vi "CAN User Interface.vi"() -> ()   [LabVIEW 2023, in "GUI.lvlib" / "Diagnostic.lvlib"]
uses:
  Diagnostic.lvlib
  Teststand Steptypes/CAN/STP/Steptypes/Control/STP Data.ctl
  HardwareAbstractionLayer_LVOOP/CAN/CAN Application Protocols/STP Protocol_class/Ctrls/STP CMD.ctl
  Teststand Steptypes/CAN/STP/Steptypes/Control/STP Out Data.ctl
  HardwareAbstractionLayer_LVOOP/CAN/CAN Application Protocols/STP Protocol_class/Ctrls/STP Error Cluster.ctl
  HardwareAbstractionLayer_LVOOP/CAN/CAN Lib/Control/CAN Table.ctl
  HardwareAbstractionLayer_LVOOP/Database/SQL Public VI/Control/DB Options.ctl
  HardwareAbstractionLayer_LVOOP/Database/Database.lvclass
  HardwareAbstractionLayer_LVOOP/CAN/CAN Lib/CAN HAL Lib.lvlib
  HardwareAbstractionLayer_LVOOP/CAN/CAN Application Protocols/STP Protocol_class/STP Protocol.lvclass
  Teststand Steptypes/LTT_TeststandSteptypes.lvlib
panel:
  in  "Socket No":u16=1
  in  "Clear":bool=TRUE
  in  "Log Data?":bool=TRUE
  out "error out":errorcluster
  in  "error in":errorcluster
  in  "Tab Control":enum32{"Query", "Logs"}(tab)
  in  "STP Data in":T1={"ECU CAN Port"="CAN1", "CMD"=130, "CAN Write Data"=[], "Response Decoder"=enum."String", "String"={"Start Index"=0, "Length"=-1}, "Number"={"MSB Index"=0, "LSB Index"=1}, "Boolean"={"Index"=0, "Bool"={"7"=FALSE, "6"=FALSE, "5"=FALSE, "4"=FALSE, "3"=FALSE, "2"=FALSE, "1"=FALSE, "0"=FALSE, "7 Enabled"=FALSE, "6 Enabled"=FALSE, "5 Enabled"=FALSE, "4 Enabled"=FALSE, "3 Enabled"=FALSE, "2 Enabled"=FALSE, "1 Enabled"=FALSE, "0 Enabled"=FALSE}}} {"CMD" items=["TSW_VERSION(130)"=130, "WAIT_EVENT(132)"=132, "SEQUENCER(133)"=133, "TSW_RESET(150)"=150, "CONFIG_ECU(151)"=151, "TEST_CORE (152)"=152, "TEST_WATCHDOG (153)"=153, "TEST_MONITORING (154)"=154, "READ_MEMORY (162)"=162, "WRITE_ERASE_MEMORY (164)"=164, "COMM_EXTERNAL (190)"=190, "COMM_INTERNAL (195)"=195, "GET_ANALOG_INPUT (210)"=210, "GET_DIGITAL_INPUT (211)"=211, "GET_FREQUENCY_INPUT (212)"=212, "TEST_INPUT_STRUCTURE (214)"=214, "GENERATE_OUTPUT_SIGNAL (220)"=220, "GENERATE_SYNCHRONIZED_OUTPUT_SIGNALS (221)"=221, "eDCU_Specific (250)"=250]; "CAN Write Data" format="%.0x"}
  out "STP Data Out":T3
  out "STP Error":T4
  out "Report Text":string
  in  "CAN View Table":T5=-1
  in  "Stop":bool caption="Blank"
  in  "Apply":bool caption="Blank"
  # "Configure STP CAN Commands"
  # "Help : the index will choose the one element in an array and compare its true or false"
  # "Bit"
  # "Value"
  # "Enabled"
  # "Help : if the LSB index is -1 then it will take only MSB value"
  # "Help : if length -1 then it will take the entire array"
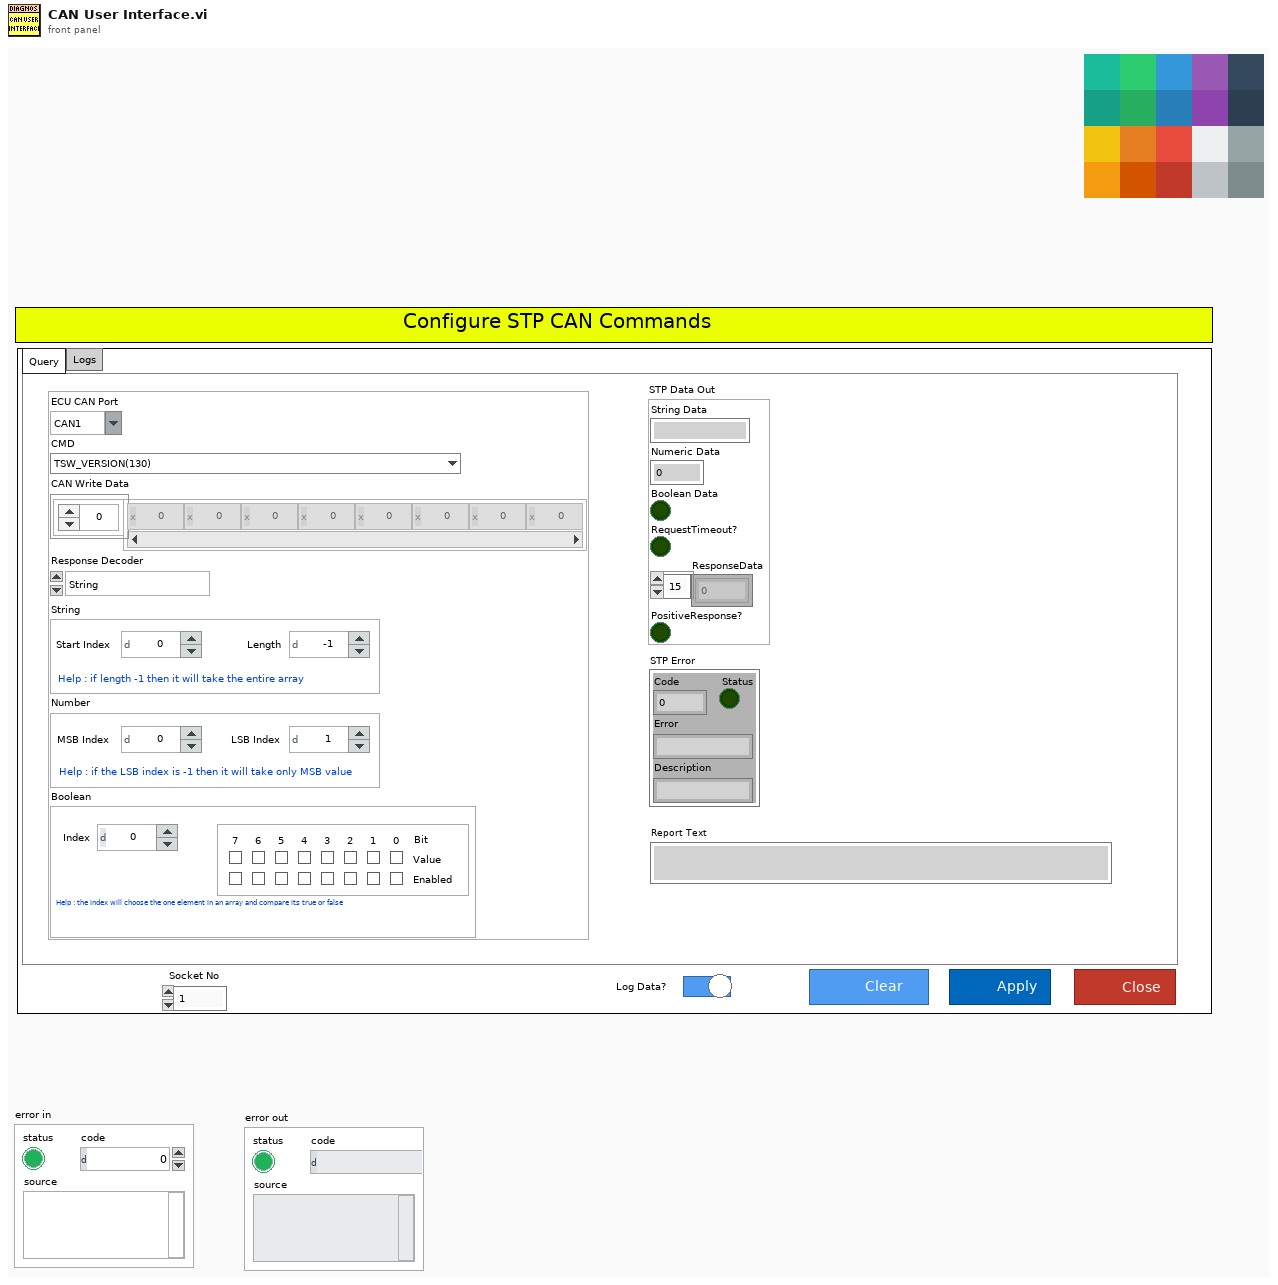
[diagram p1: front panel]
types:
  T1 = typedef "LTT_TeststandSteptypes.lvlib/STP Data.ctl" = cluster{"ECU CAN Port":string, "CMD":T2, "CAN Write Data":u8[], "Response Decoder":enum16{"String", "Number", "Boolean"}, "String":cluster{"Start Index":i32, "Length":i32}, "Number":cluster{"MSB Index":i32, "LSB Index":i32}, "Boolean":cluster{"Index":i32, "Bool":cluster{"7":bool, "6":bool, "5":bool, "4":bool, "3":bool, "2":bool, "1":bool, "0":bool, "7 Enabled":bool, "6 Enabled":bool, "5 Enabled":bool, "4 Enabled":bool, "3 Enabled":bool, "2 Enabled":bool, "1 Enabled":bool, "0 Enabled":bool}}}
  T2 = typedef "HardwareAbstractionLayer_LVOOP.lvlib/CAN Application Protocols Lib.lvlib/STP Protocol.lvclass/STP CMD.ctl" = u8
  T3 = typedef "LTT_TeststandSteptypes.lvlib/STP Out Data.ctl" = cluster{"String Data":string, "Numeric Data":dbl, "Boolean Data":bool, "RequestTimeout?":bool, "ResponseData":u8[], "PositiveResponse?":bool}
  T4 = typedef "HardwareAbstractionLayer_LVOOP.lvlib/CAN Application Protocols Lib.lvlib/STP Protocol.lvclass/STP Error Cluster.ctl" = cluster{"Status":bool, "Code":u8, "Error":string, "Description":string}
  T5 = typedef "HardwareAbstractionLayer_LVOOP.lvlib/CAN HAL Lib.lvlib/CAN Table.ctl" = i32
  T6 = typedef "HardwareAbstractionLayer_LVOOP.lvlib/Database.lvclass/DB Options.ctl" = enum16{"Init", "Select Data", "Insert Data", "Update Data", "Delete Data", "Execute Query", "Create Schema", "Create Table", "List Tables", "List Columns", "Close"}
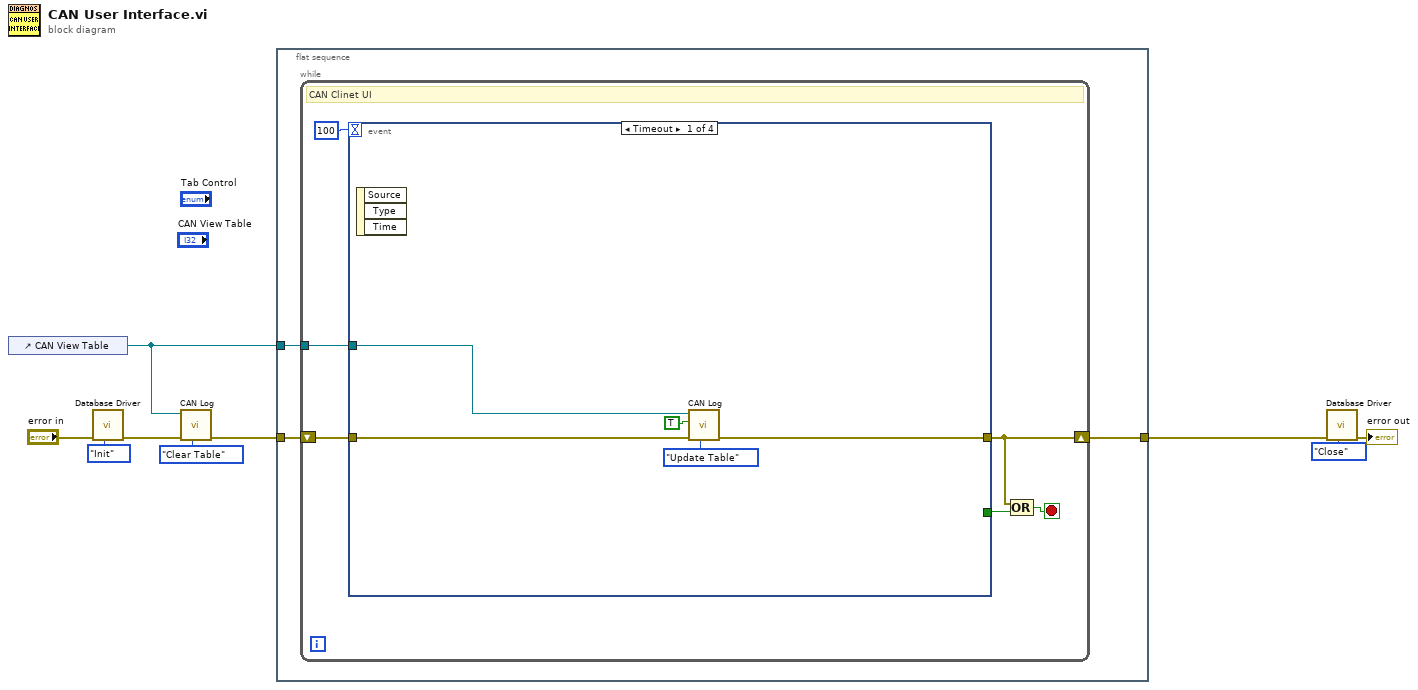
[diagram p0: block diagram]
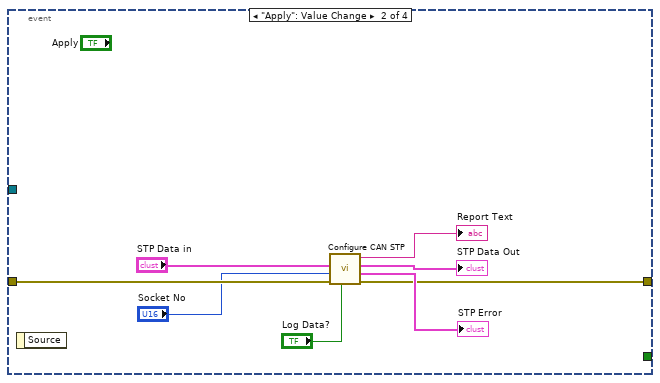
[diagram p2: hidden frame]
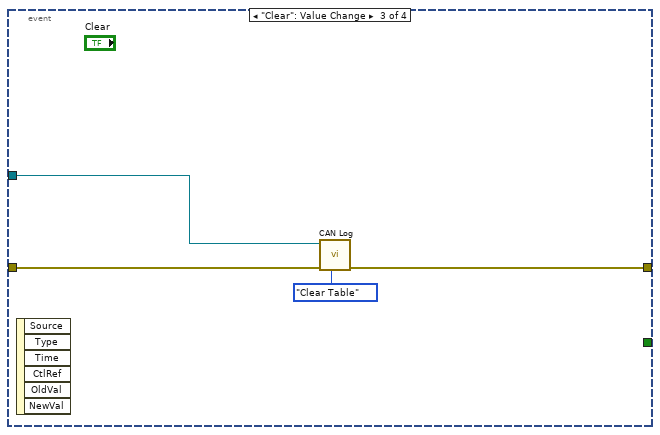
[diagram p3: hidden frame]
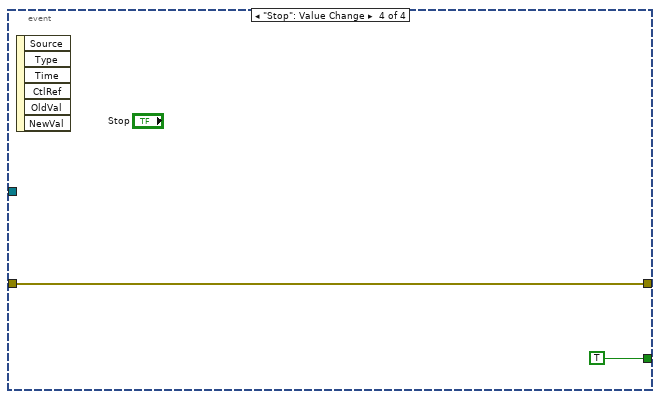
[diagram p4: hidden frame]
diagram:
  n1 = control-ref of="CAN View Table"() -> (w1:refnum<vi>)
  n2 = call "Database Driver.vi"("Options"=DB_Options."Init", "error in"="error in") -> ("error out"=w3:errorcluster)  [unwired: 6 in, 3 out]
  n3 = call "CAN Log.vi"("Action"=enum16{"Update Table", "Clear Table"}."Clear Table", "error in (no error)"=w3, "CAN View Table"=w1) -> ("error out"=w2:errorcluster)  [unwired: 7 in, 1 out]
  n4 = flat-sequence {
    tunnel: [w11] -> w7
    tunnel: w2 -> [w12]
    tunnel: w1 -> [w10]
    frame #0 {
      n5 = while {
        tunnel: w10 -> [w15]
        shift-right: [w13] -> w11
        shift-left: w12 -> [w16]
        stop <- w14 stop-if-true
        # "CAN Clinet UI"
        n6 = event shown="[0] Timeout" {
          selector: _ -> [_ _ _ _]
          dyn-events: _ -> [_ _ _ _]
          timeout: 100 -> [_ _ _ _]
          tunnel: [_ _ _ TRUE] -> w17
          tunnel: w16 -> [w22 w30 w35 w36]
          tunnel: [w20 w24 w34 w36] -> w13
          tunnel: w15 -> [w21 _ w32 _]
          event Timeout {
            n7 = event-data() -> ()  [unwired: 1 in, 3 out]
            n8 = call "CAN Log.vi"("Action"=enum16{"Update Table", "Clear Table"}."Update Table", "error in (no error)"=w22, "Hexadecimal?"=TRUE, "CAN View Table"=w21) -> ("error out"=w20:errorcluster)  [unwired: 6 in, 1 out]
          }
          event "Apply": Value Change {
            n9 = event-data() -> ()  [unwired: 1 in, 1 out]
            n10 = call "Configure CAN STP.vi"("Log Data?"="Log Data?", "error in"=w30, "Socket No"="Socket No", "STP Data in"="STP Data in") -> ("error out"=w24:errorcluster, "STP Error"=→"STP Error":T4, "STP Data Out"=→"STP Data Out":T3, "Report Text"=→"Report Text":string)  [unwired: 4 in]
          }
          event "Clear": Value Change {
            n11 = event-data() -> ()  [unwired: 1 in, 6 out]
            n12 = call "CAN Log.vi"("Action"=enum16{"Update Table", "Clear Table"}."Clear Table", "error in (no error)"=w35, "CAN View Table"=w32) -> ("error out"=w34:errorcluster)  [unwired: 7 in, 1 out]
          }
          event "Stop": Value Change {
            n13 = event-data() -> ()  [unwired: 1 in, 6 out]
          }
        }
        n14 = Compound Arithmetic op=OR(w13, w17) -> (w14:bool)
      }
    }
  }
  n15 = call "Database Driver.vi"("Options"=DB_Options."Close", "error in"=w7) -> ("error out"=→"error out":errorcluster)  [unwired: 6 in, 3 out]
